vi "Configure Sequencer List Current Index.vi"(8 "error in (no error)":errorcluster, 9 "Current Index (0)":i32, 10 "Instance (1)":i32=1, 11 "VISA resource name":refnum<visa-resource-name>) -> (0 "error out":errorcluster, 3 "VISA resource name out":refnum<visa-resource-name>)   [LabVIEW 2015, in "Rohde&Schwarz CMXP GPRF.lvlib"]
doc: "Selects an entry of the sequencer list. Some other properties use this setting.\n\nAttribute:\nRSCMXPGPRF_ATTR_SEQUENCER_LIST_CURRENT_INDEX\n\nRemote-control command:\nSOURce:GPRF:GEN<i>:SEQuencer:LIST:INDex"
uses:
  <instrlib>/Rohde&Schwarz CMXP GPRF/Rohde&Schwarz CMXP GPRF.lvlib
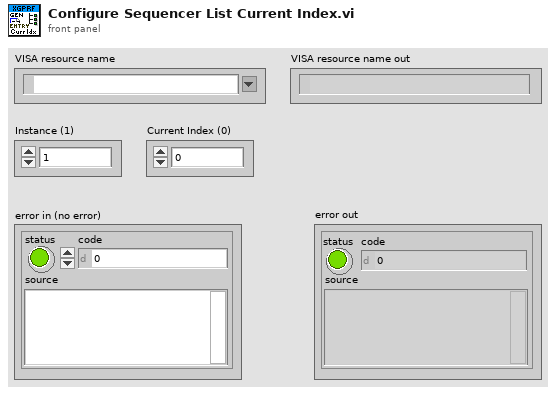
[diagram p1: front panel]
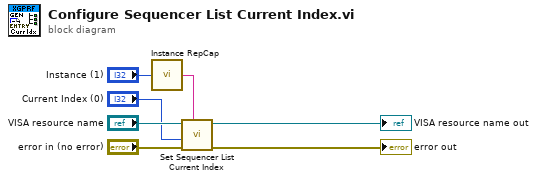
[diagram p0: block diagram]
diagram:
  n1 = call <instrlib>:"Instance RepCap.vi"("instance  in"="Instance (1)") -> ("instance out"=w2:string)
  n2 = call "Set Sequencer List Current Index"("Repeated Capabilities"=w2, "error in (no error)"="error in (no error)", "Sequencer List Current Index (0)"="Current Index (0)", "instrument handle"="VISA resource name") -> ("error out"=→"error out":errorcluster, "instrument handle out"=→"VISA resource name out":refnum<visa-resource-name>)  [unwired: 6 in]
